vi "PrintTemperature.vi"(8 "error in (no error)":errorcluster, 10 "Address":u8=1 min=1, 11 "VISA resource name":refnum<visa-resource-name>) -> (0 "error out":errorcluster, 1 "Raw Response":string, 2 "Temperature":dbl, 3 "VISA resource name out":refnum<visa-resource-name>)   [LabVIEW 2020, in "driver_flodx_pressure.lvlib"]
uses:
  <instrlib>/RxnRover/FloDx Pressure Driver/driver_flodx_pressure.lvlib
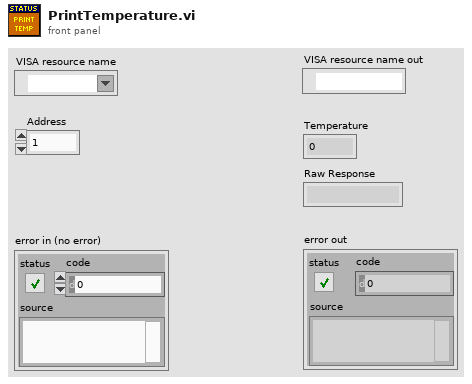
[diagram p1: front panel]
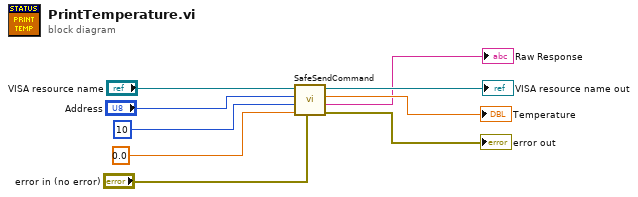
[diagram p0: block diagram]
diagram:
  n1 = call <instrlib>:"SafeSendCommand.vi"("error in"="error in (no error)", "Parameter"=sgl 0.0 ("Parameter(float)"), "Command #"=u8 10 ("Command"), "Address #"="Address", "VISA resource name"="VISA resource name") -> ("error out"=→"error out":errorcluster, "Raw Response"=→"Raw Response":string, "Value"=→"Temperature":dbl, "VISA resource name out"=→"VISA resource name out":refnum<visa-resource-name>)  [unwired: 3 in]
